vi "Translator.StrictTypeDefCheck.vi"(8 "error in (no error)":errorcluster, 11 "Ctl Refnum in":refnum<vi>) -> (0 "error out":errorcluster, 2 "Strict Type def?":bool, 3 "Ctl Refnum out":refnum<vi>)   [LabVIEW 2019, in "Tools.lvlib"]
uses:
  Tools.lvlib
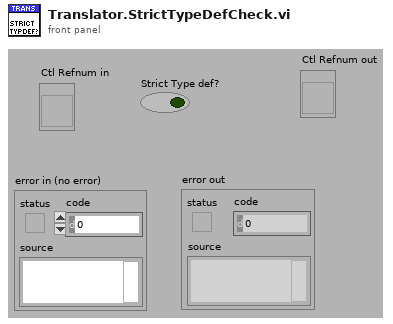
[diagram p1: front panel]
types:
  T1 = enum32{"not a typedef", "typedef", "strict typedef"}
  T2 = enum32{"not a typedef", "typedef", "strict typedef", "class private data"}
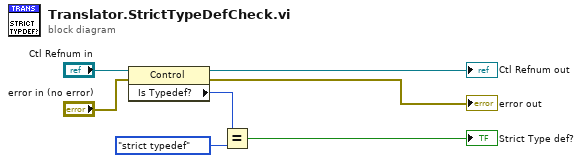
[diagram p0: block diagram]
diagram:
  n1 = property class="Control"(reference="Ctl Refnum in", error in="error in (no error)") -> (reference out=→"Ctl Refnum out":refnum<vi>, error out=→"error out":errorcluster, "Is Typedef?"=w3:T2)
  n2 = Equal?(x=w3, y=T1."strict typedef" ("Is Typedef?")) -> (x = y?=→"Strict Type def?":bool)
